vi "Agilent PSG MXG_Open.vi"(8 "error in":errorcluster, 10 "Reset?":bool=TRUE, 11 "Alias":string) -> (0 "error out":errorcluster {"code" format="%.0x"}, 3 "Handle":variant)   [LabVIEW 2015]
uses:
  <instrlib>/Agilent PSG MXG Series/Agilent PSG MXG Series.lvlib
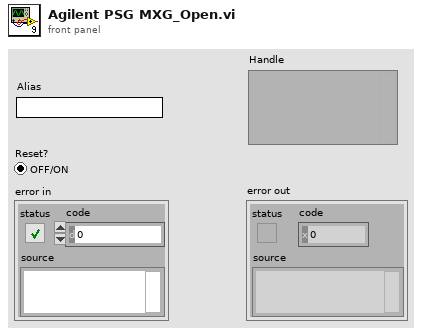
[diagram p1: front panel]
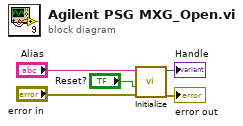
[diagram p0: block diagram]
diagram:
  n1 = call <instrlib>:"Initialize.vi"("error in (no error)"="error in", "Reset (True)"="Reset?", "VISA resource name"="Alias") -> ("error out"=→"error out":errorcluster, "VISA resource name out"=→"Handle":refnum<visa-resource-name>)  [unwired: 7 in]
